vi "KE6485GUI.constructor.vi"(0 "name":string, 2 "data in":string, 5 "error in (no error)":errorcluster) -> (14 "i ref out":refnum<vi>, 16 "data out":string, 19 "error out":errorcluster)   [LabVIEW 2014, in "KE6485GUI.lvlib"]
doc: "This is the constructor of a class.\n\nLicense Agreement for this software:\n\nCopyright (C)\nGesellschaft für Schwerionenforschung, GSI\nPlanckstr. 1\n64291 Darmstadt\nGermany\n\nContact: D.Beck@gsi.de \n\nThis program is free software; you can redistribute it and/or modify it under the terms of the GNU General Public License as published by the Free Software Foundation; either version 2 of the license, or (at your option) any later version.\n\nThis program is distributed in the hope that it will be useful, but WITHOUT ANY WARRANTY; without even the implied warranty of MERCHANTABILITY or FITNESS FOR A PARTICULAR PURPOSE. See the GNU General License for more details (http://www.gnu.org).\n\nGesellschaft für Schwerionenforschung, GSI\nPlanckstr. 1, 64291 Darmstadt, Germany\nFor all questions and ideas contact: M.Richter@gsi.de, H.Brand@gsi.de or D.Beck@gsi.de.\nLast update: 17-JUN-2004"
uses:
  KE6485GUI.lvlib
  CSlibraries-extern/DimLVEvent/LVDimInterface/LVDimInterface.dis_add_command_notifier.vi
  CSCore/CSSystem/CSSystemLib/CSSystemLib.lvlib
  CSCore/GUIs/GOGUserGUIs/DeviceBaseGUI/DeviceBaseGUI.lvlib
  CSlibraries-extern/DimLVEvent/LVDimInterface/LVDimInterface.lvlib
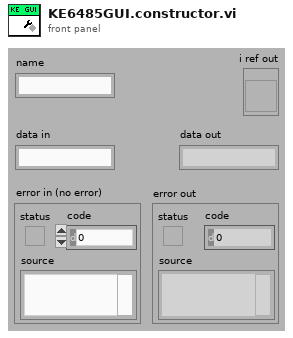
[diagram p1: front panel]
types:
  T1 = enum16{"SetAttribute", "GetAttribute", "CreateAttribute", "DestroyAttribute", "DestroyAllAtributes"}
  T2 = typedef "DeviceBaseGUI.lvlib/DeviceBaseGUI.i attribute.ctl" = cluster{"GOGFrontPanel.i attribute":T3}
  T3 = typedef "GOGFrontPanel.lvlib/GOGFrontPanel.i attribute.ctl" = cluster{"GOGObject":string, "Object":string, "Method":string, "Descriptor":T4, "Input Descriptor":string, "Output Descriptor":string, "inputNames":string[], "outputNames":string[], "Values":cluster{"descriptor":string, "value":string}[]}
  T4 = typedef "BaseProcess.lvlib/BaseProcess.descriptor string definition.ctl" = string
  T5 = cluster{"commandID":i32, "notifier out":refnum<notifier>}
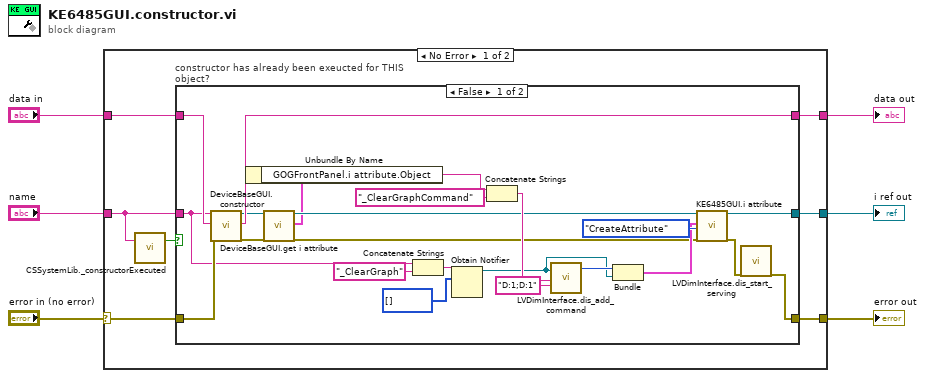
[diagram p0: block diagram]
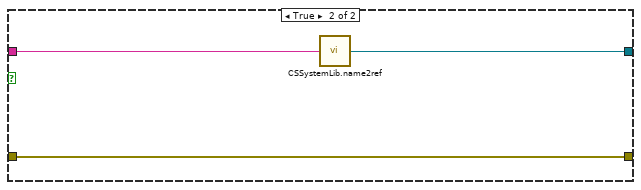
[diagram p2: hidden frame]
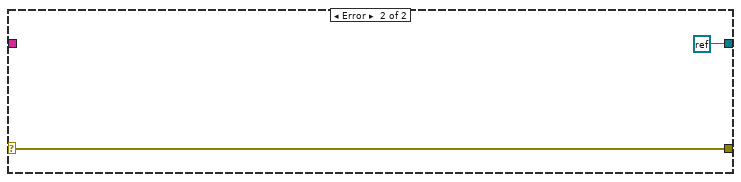
[diagram p3: hidden frame]
diagram:
  n1 = case shown="No Error" "error in (no error)" {
    selector: "error in (no error)" -> [w11 w40]
    tunnel: [w13 refnum<k0> refnum] -> w6
    tunnel: [w12 w40] -> w5
    tunnel: "name" -> [w9 _]
    tunnel: "data in" -> [w8 _]
    tunnel: [w7 _] -> w1
    frame No Error {
      n2 = call "CSSystemLib._constructorExecuted.vi"("name"=w9) -> ("constructor executed?"=w10:bool)  [unwired: 18 in]
      n3 = case "constructor has already been exeucted for THIS object?" shown="False" w10 {
        tunnel: [w35 w38] -> w13
        tunnel: [w21 w37] -> w12
        tunnel: w9 -> [w27 w39]
        tunnel: w11 -> [w34 w37]
        tunnel: w8 -> [w31 _]
        tunnel: [w33 _] -> w7
        frame False {
          n4 = call "DeviceBaseGUI.constructor.vi"("name"=w27, "data in"=w31, "error in (no error)"=w34) -> ("i ref out"=w17:refnum<vi>, "data out"=w33:string, "error out"=w19:errorcluster)  [unwired: 14 in]
          n5 = call "DeviceBaseGUI.get i attribute.vi"("i ref in"=w17, "error in (no error)"=w19) -> ("i ref out"=w16:refnum<vi>, "i attribute"=w15:T2, "error out"=w18:errorcluster)  [unwired: 15 in]
          n6 = Unbundle By Name(w15) -> ("GOGFrontPanel.i attribute.Object"=w14:string)
          n7 = Concatenate Strings(w27, "_ClearGraph" ("string")) -> (w32:string)
          n8 = Obtain Notifier(name (unnamed)=w32, notification data type=i8[] []) -> (notifier out=w20:refnum<notifier>)  [unwired: 2 in, 2 out]
          n9 = Concatenate Strings(w14, "_ClearGraphCommand" ("string")) -> (w26:string)
          n10 = call-poly "LVDimInterface.dis_add_command.vi"("notifier"=w20, "commandName"=w26, "typeDescriptor"="D:1;D:1") -> ("commandID"=w24:i32)  [unwired: 15 in, 1 out]
          n11 = Bundle("commandID"=w24, "notifier out"=w20) -> (w23:T5)  [unwired: 1 in]
          n12 = call "KE6485GUI.i attribute.vi"("VI Refnum"=w16, "CLASS.i attribute"=w23, "Action"=T1."CreateAttribute", "error in (no error)"=w18) -> ("VI Refnum out"=w35:refnum<vi>, "error out"=w22:errorcluster)  [unwired: 13 in, 1 out]
          n13 = call "LVDimInterface.dis_start_serving.vi"("error in (no error)"=w22) -> ("error out"=w21:errorcluster)  [unwired: 17 in, 1 out]
        }
        frame True {
          n14 = call "CSSystemLib.name2ref.vi"("name"=w39) -> ("obj refnum"=w38:refnum<vi>)
        }
      }
    }
    frame Error {
    }
  }
  "i ref out" <- w6
  "error out" <- w5
  "data out" <- w1
